vi "Kelompok 3_While Loop.vi"() -> ()   [LabVIEW 2020]
panel:
  in  "input 3":dbl
  out "output 3":dbl
  out "output 2":dbl
  in  "input 2":dbl
  in  "stop":bool
  out "True/False":bool
  out "output":dbl
  in  "input":dbl
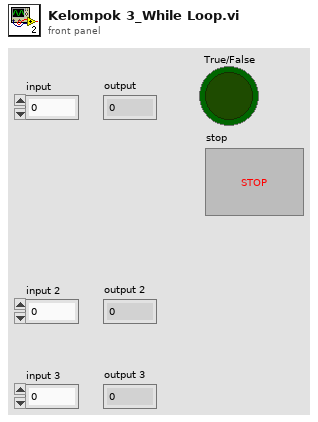
[diagram p1: front panel]
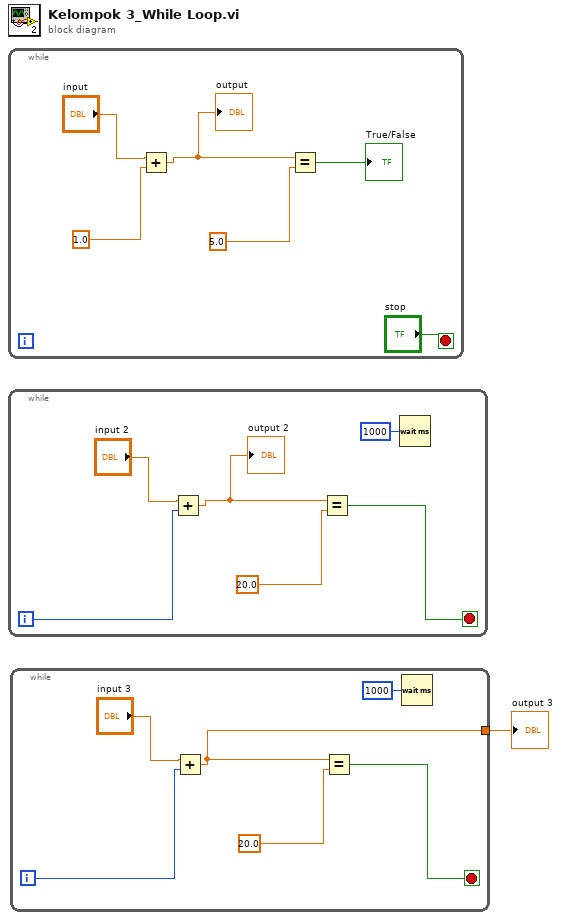
[diagram p0: block diagram]
diagram:
  n1 = while {
    stop <- "stop" stop-if-true
    n2 = Add(x="input", y=1.0) -> (x+y=w6:dbl)
    "output" <- w6
    n3 = Equal?(x=w6, y=5.0) -> (x = y?=→"True/False":bool)
  }
  n4 = while {
    i -> [w10]
    stop <- w9 stop-if-true
    n5 = Add(x="input 2", y=w10) -> (x+y=w12:dbl)
    "output 2" <- w12
    n6 = Equal?(x=w12, y=20.0) -> (x = y?=w9:bool)
    n7 = Wait (ms)(milliseconds to wait=u32 1000) -> ()  [unwired: 1 out]
  }
  n8 = while {
    tunnel: [w14] -> w1
    i -> [w17]
    stop <- w16 stop-if-true
    n9 = Add(x="input 3", y=w17) -> (x+y=w14:dbl)
    n10 = Equal?(x=w14, y=20.0) -> (x = y?=w16:bool)
    n11 = Wait (ms)(milliseconds to wait=u32 1000) -> ()  [unwired: 1 out]
  }
  "output 3" <- w1
